vi "Begin.vi"(8 "error in (no error)":errorcluster, 10 "Settings":variant, 11 "Elevator Concrete in":refnum<class "Elevator Linear.lvclass">) -> (0 "error out":errorcluster, 3 "Elevator Concrete out":refnum<class "Elevator Linear.lvclass">)   [LabVIEW 2019, in "Elevator.lvlib" / "Elevator Linear.lvclass"]
doc: "This VI intializes the linear elevator."
uses:
  Elevator Linear.lvclass
  C:/Users/Public/Documents/2020InfinteRecharge/src robot/Classes/Elevator/Elevator.lvclass
  <vilib>/Rock Robotics/WPI/ThirdParty/Phoenix-LabVIEW/Motor Controller/Controls/CTRE_Phoenix_MotorControl_EnhancedMotorControllerConfigurables.ctl
  <vilib>/Rock Robotics/WPI/ThirdParty/Phoenix-LabVIEW/Motor Controller/Controls/CTRE_Phoenix_MotorControl_BaseConfigurables.ctl
  <vilib>/Rock Robotics/WPI/ThirdParty/Phoenix-LabVIEW/Motor Controller/Controls/CTRE_Phoenix_MotorControl_VelocityMeasurementPeriod.ctl
  <vilib>/Rock Robotics/WPI/ThirdParty/Phoenix-LabVIEW/Motor Controller/Controls/CTRE_Phoenix_MotorControl_SlotStructure.ctl
  <vilib>/Rock Robotics/WPI/ThirdParty/Phoenix-LabVIEW/Motor Controller/Controls/CTRE_Phoenix_MotorControl_FilterStruct.ctl
  <vilib>/Rock Robotics/WPI/ThirdParty/Phoenix-LabVIEW/Motor Controller/Controls/CTRE_Phoenix_MotorControl_RemoteSourceType.ctl
  <vilib>/Rock Robotics/WPI/ThirdParty/Phoenix-LabVIEW/Controls/CTRE_Phoenix_CustomParamConfiguration.ctl
  <vilib>/Rock Robotics/WPI/ThirdParty/Phoenix-LabVIEW/Motor Controller/Controls/CTRE_Phoenix_MotorControl_FeedbackDevice.ctl
  <vilib>/Rock Robotics/WPI/ThirdParty/Phoenix-LabVIEW/Motor Controller/Controls/CTRE_Phoenix_MotorControl_SensorTermFeedbackDevice_Enhanced.ctl
  <vilib>/Rock Robotics/WPI/ThirdParty/Phoenix-LabVIEW/Motor Controller/Controls/CTRE_Phoenix_MotorControl_LimitSwitchNormal.ctl
  <vilib>/Rock Robotics/WPI/ThirdParty/Phoenix-LabVIEW/Motor Controller/Controls/CTRE_Phoenix_MotorControl_LimitSwitchSource_Local.ctl
  Controls/Elevator Position.ctl
  Elevator Linear.lvclass/Elevator Linear.ctl
  Elevator.lvclass/Elevator.ctl
  Public Methods/Read Elevator Linear PID.vi
  Public Methods/Write Array.vi
  <vilib>/Rock Robotics/WPI/ThirdParty/Phoenix-LabVIEW/Motor Controller/Get/CTRE_Phoenix_MotorController_GetLimitSwitchStates.vi
  Elevator.lvclass
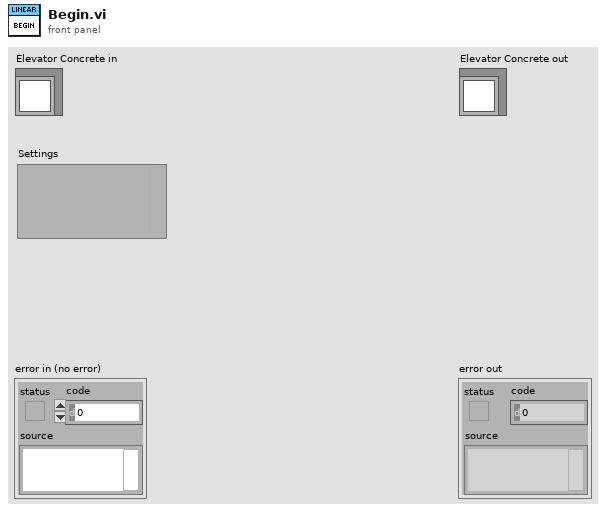
[diagram p1: front panel]
types:
  T1 = typedef "Elevator.lvlib/Elevator.lvclass/Elevator Position.ctl" = enum16{"CS, Cargo Ship Cargo", "C0, Cargo Ground", "C1, LV1 Cargo", "C2, LV2 Cargo", "C3, LV3 Cargo", "H0, LV1 Hatch", "H1, LV2 Hatch", "H2, LV3 Hatch"}
  T2 = enum16{"FollowerType_PercentOutput", "FollowerType_AuxOutput1"}
  T3 = typedef "CTRE_Phoenix_MotorControl_EnhancedMotorControllerConfigurables.ctl" = cluster{"Base Configurables":T4, "primaryPID":cluster{"selectedFeedbackCoefficient":dbl, "selectedFeedbackSensor":T10}, "auxiliaryPID":cluster{"selectedFeedbackCoefficient":dbl, "selectedFeedbackSensor":T10}, "sum0Term":T11, "sum1Term":T11, "diff0Term":T11, "diff1Term":T11, "forwardLimitSwitchNormal":T12, "reverseLimitSwitchNormal":T12, "forwardLimitSwitchDeviceID":i32, "reverseLimitSwitchDeviceID":i32, "forwardLimitSwitchSource":T13, "reverseLimitSwitchSource":T13, "peakCurrentLimit":i32, "peakCurrentDuration":i32, "continuousCurrentLimit":i32}
  T4 = typedef "CTRE_Phoenix_MotorControl_BaseConfigurables.ctl" = cluster{"openLoopRamp":dbl, "closedLoopRamp":dbl, "peakOutputForward":dbl, "peakOutputReverse":dbl, "nominalOutputForward":dbl, "nominalOutputReverse":dbl, "neutralDeadband":dbl, "voltageCompSaturation":dbl, "voltageMeasurementFilter":i32, "velocityMeasurementPeriod":T5, "velocityMeasurementWindow":i32, "forwardSoftLimitThreshold":i32, "reverseSoftLimitThreshold":i32, "forwardSoftLimitEnable":bool, "reverseSoftLimitEnable":bool, "slot0":T6, "slot1":T6, "slot2":T6, "slot3":T6, "auxPIDPolarity":bool, "remoteFilter0":T7, "remoteFilter1":T7, "motionCruiseVelocity":i32, "motionAcceleration":i32, "motionProfileTrajectoryPeriod":i32, "feedbackNotContinuous":bool, "remoteSensorClosedLoopDisableNeutralOnLOS":bool, "clearPositionOnLimitF":bool, "clearPositionOnLimitR":bool, "clearPositionOnQuadIdx":bool, "limitSwitchDisableNeutralOnLOS":bool, "softLimitDisableNeutralOnLOS":bool, "pulseWidthPeriod_EdgesPerRot":i32, "pulseWidthPeriod_FilterWindowSz":i32, "customParam":T9, "trajectoryInterpolationEnable":bool}
  T5 = typedef "CTRE_Phoenix_MotorControl_VelocityMeasurementPeriod.ctl" = u16
  T6 = typedef "CTRE_Phoenix_MotorControl_SlotStructure.ctl" = cluster{"P":dbl, "I":dbl, "D":dbl, "F":dbl, "integralZone":dbl, "allowableClosedLoopError":i32, "maxIntegralAccumulator":dbl, "closedLoopPeakOutput":dbl, "closedLoopPeriod":i32}
  T7 = typedef "CTRE_Phoenix_MotorControl_FilterStruct.ctl" = cluster{"remoteSensorDeviceID":u8, "remoteSensorSource":T8}
  T8 = typedef "CTRE_Phoenix_MotorControl_RemoteSourceType.ctl" = enum16{"Off", "Talon SRX Selected Sensor", "Pigeon IMU Yaw", "Pigeon IMU Pitch", "Pigeon IMU Roll", "CANifier Quadrature", "CANifier PWM Input 0", "CANifier PWM Input 1", "CANifier PWM Input 2", "CANifier PWM Input 3", "Gadgeteer Pigeon Yaw", "Gadgeteer Pigeon Pitch", "Gadgeteer Pigeon Roll", "CANCoder"}
  T9 = typedef "CTRE_Phoenix_CustomParamConfiguration.ctl" = cluster{"customParam0":i32, "customParam1":i32}
  T10 = typedef "CTRE_Phoenix_MotorControl_FeedbackDevice.ctl" = i8
  T11 = typedef "CTRE_Phoenix_MotorControl_SensorTermFeedbackDevice_Enhanced.ctl" = i8
  T12 = typedef "CTRE_Phoenix_MotorControl_LimitSwitchNormal.ctl" = enum16{"Normally Open", "Normally Closed", "Disabled"}
  T13 = typedef "CTRE_Phoenix_MotorControl_LimitSwitchSource_Local.ctl" = enum16{"Feedback Connector", "Remote Talon SRX", "Remote CANifier", "Deactivated"}
  T14 = typedef "Elevator.lvlib/Elevator.lvclass/Elevator Constants.ctl" = cluster{"Arm Motion Magic Max Velocity":u32, "Arm Motion Magic Max Acceleration":u32, "Wrist Motion Magic Max Velocity":u32, "Wrist Motion Magic Max Acceleration":u32, "Elevator Linear Motion Magic Max Velocity":u32, "Elevator Linear Motion Magic Max Acceleration":u32, "Arm Gear Ratio":dbl, "Wrist Gear Ratio":dbl, "Elevator Linear Gear Ratio":dbl, "Arm Encoder ABS Value":i32, "Wrist Encoder ABS Value":i32}
  T15 = typedef "Elevator.lvlib/Elevator.lvclass/Elevator IDs.ctl" = cluster{"Wrist":u8, "Left Master":u8, "Left Slave":u8, "Right Master":u8, "Right Slave":u8, "Vacumm Pump 1":u8, "Vacumm Pump 2":u8, "Elevator Linear Master":u8, "Elevator Linear Slave":u8}
  T16 = typedef "WPI_MotorControlDeviceRef.ctl" = cluster{"DeviceStatus":errorcluster, "Type":T17, "PWM":cluster{"PWM Channel":T18, "DeadBand":T19}, "CAN":cluster{"Device Number":u8, "SetOutput VI Ref":variant, "GetOutput VI Ref":variant, "Enable VI Ref":variant, "Disable VI Ref":variant, "Data":variant}, "Invert":bool, "DIO PWM":cluster{"PWM \"Enable\" Channel":T18, "DIOChannel":T20, "PWM Rate":dbl}}
  T17 = typedef "WPI_MotorControlType.ctl" = enum16{"PWM", "CAN", "DIO PWM"}
  T18 = typedef "FPGA_DIOPWMChannel.ctl" = enum8{"PWM 0", "PWM 1", "PWM 2", "PWM 3", "PWM 4", "PWM 5", "PWM 6", "PWM 7", "PWM 8", "PWM 9", "PWM MXP 0", "PWM MXP 1", "PWM MXP 2", "PWM MXP 3", "PWM MXP 4", "PWM MXP 5", "PWM MXP 6", "PWM MXP 7", "PWM MXP 8", "PWM MXP 9", "Invalid"}
  T19 = typedef "WPI_PWMDeadband.ctl" = cluster{"Name":string, "maxPositivePwm":i32, "minPositivePwm":i32, "centerPwm":i32, "maxNegativePwm":i32, "minNegativePwm":i32, "angularRange":u16}
  T20 = typedef "FPGA_DIOChannel.ctl" = enum8{"DIO 0", "DIO 1", "DIO 2", "DIO 3", "DIO 4", "DIO 5", "DIO 6", "DIO 7", "DIO 8", "DIO 9", "DIO MXP 0", "DIO MXP 1", "DIO MXP 2", "DIO MXP 3", "DIO MXP 4", "DIO MXP 5", "DIO MXP 6", "DIO MXP 7", "DIO MXP 8", "DIO MXP 9", "DIO MXP 10", "DIO MXP 11", "DIO MXP 12", "DIO MXP 13", "DIO MXP 14", "DIO MXP 15", "SPI Port CS1", "SPI Port CS2", "SPI Port CS3", "SPI Port MISO", "SPI Port MOSI", "Invalid"}
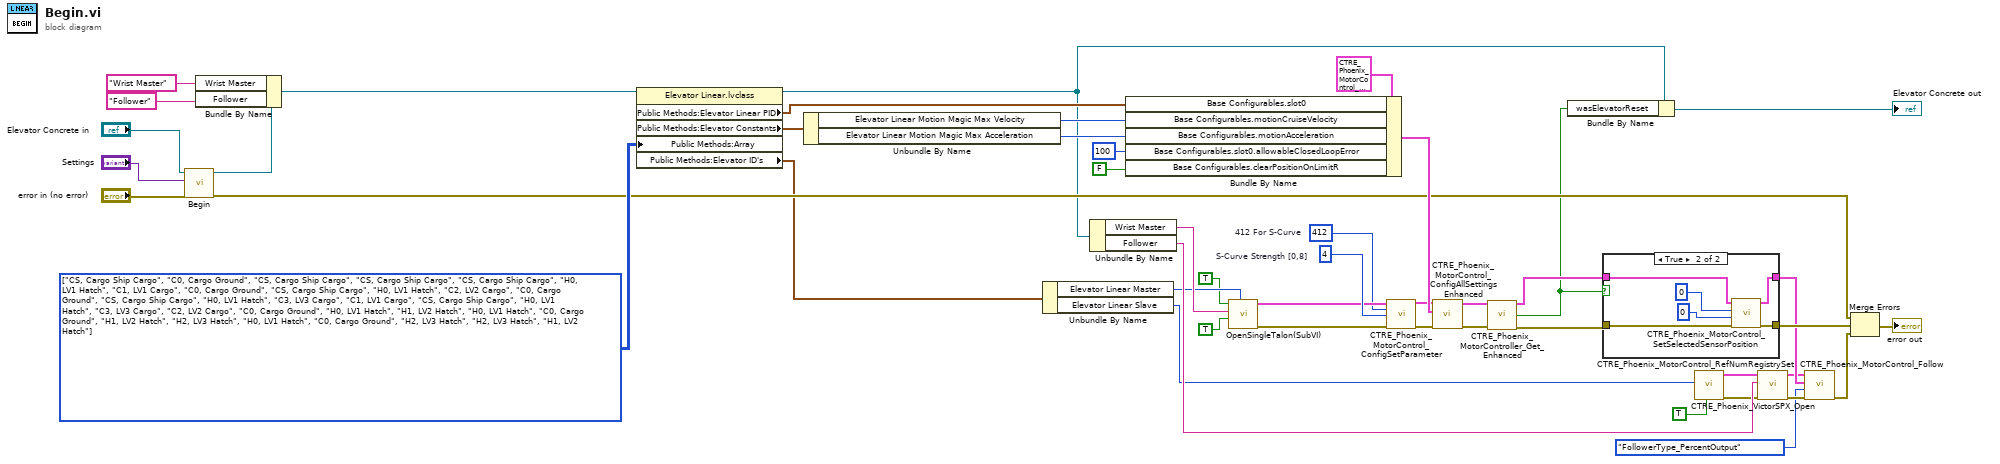
[diagram p0: block diagram]
diagram:
  w17 = T1[][] [[enum."CS, Cargo Ship Cargo", enum."C0, Cargo Ground", enum."CS, Cargo Ship Cargo", enum."CS, Cargo Ship Cargo"], [enum."CS, Cargo Ship Cargo", enum."H0, LV1 Hatch", enum."C1, LV1 Cargo", enum."C0, Cargo Ground"], [enum."CS, Cargo Ship Cargo", enum."H0, LV1 Hatch", enum."C2, LV2 Cargo", enum."C0, Cargo Ground"], [enum."CS, Cargo Ship Cargo", enum."H0, LV1 Hatch", enum."C3, LV3 Cargo", enum."C1, LV1 Cargo"], [enum."CS, Cargo Ship Cargo", enum."H0, LV1 Hatch", enum."C3, LV3 Cargo", enum."C2, LV2 Cargo"], [enum."C0, Cargo Ground", enum."H0, LV1 Hatch", enum."H1, LV2 Hatch", enum."H0, LV1 Hatch"], [enum."C0, Cargo Ground", enum."H1, LV2 Hatch", enum."H2, LV3 Hatch", enum."H0, LV1 Hatch"], [enum."C0, Cargo Ground", enum."H2, LV3 Hatch", enum."H2, LV3 Hatch", enum."H1, LV2 Hatch"]] items=["CS, Cargo Ship Cargo", "C0, Cargo Ground", "C1, LV1 Cargo", "C2, LV2 Cargo", "C3, LV3 Cargo", "H0, LV1 Hatch", "H1, LV2 Hatch", "H2, LV3 Hatch"] ("Array")
  w32 = u32 412  # 412 For S-Curve
  w37 = 4  # S-Curve Strength [0,8]
  n1 = call-parent "Begin.vi"("error in (no error)"="error in (no error)", "Settings"="Settings", "Elevator in"="Elevator Concrete in") -> ("error out"=w12:errorcluster, "Elevator out"=w14:refnum<class "Elevator Linear.lvclass">)  [unwired: 7 in]
  n2 = Bundle By Name(cluster=w14, "Wrist Master"="Wrist Master", "Follower"="Follower") -> (w28:refnum<class "Elevator Linear.lvclass">)
  n3 = property class="Elevator Linear.lvclass"(reference=w28, "Public Methods:Array"=w17) -> (reference out=w4:refnum<class "Elevator Linear.lvclass">, "Public Methods:Elevator Linear PID"=w11:T6, "Public Methods:Elevator Constants"=w18:T14, "Public Methods:Elevator ID's"=w5:T15)  [unwired: 1 in, 1 out]
  n4 = Unbundle By Name(w18) -> ("Elevator Linear Motion Magic Max Velocity"=w41:u32, "Elevator Linear Motion Magic Max Acceleration"=w40:u32)
  n5 = Unbundle By Name(w5) -> ("Elevator Linear Master"=w38:u8, "Elevator Linear Slave"=w39:u8)
  n6 = Unbundle By Name(w4) -> ("Wrist Master"=w46:string, "Follower"=w45:string)
  n7 = Bundle By Name(cluster=T3 {"Base Configurables"={"openLoopRamp"=0.0, "closedLoopRamp"=0.0, "peakOutputForward"=1.0, "peakOutputReverse"=-1.0, "nominalOutputForward"=0.0, "nominalOutputReverse"=0.0, "neutralDeadband"=0.04, "voltageCompSaturation"=0.0, "voltageMeasurementFilter"=32, "velocityMeasurementPeriod"=100, "velocityMeasurementWindow"=64, "forwardSoftLimitThreshold"=0, "reverseSoftLimitThreshold"=0, "forwardSoftLimitEnable"=FALSE, "reverseSoftLimitEnable"=FALSE, "slot0"={"P"=0.0, "I"=0.0, "D"=0.0, "F"=0.0, "integralZone"=0.0, "allowableClosedLoopError"=0, "maxIntegralAccumulator"=0.0, "closedLoopPeakOutput"=1.0, "closedLoopPeriod"=1}, "slot1"={"P"=0.0, "I"=0.0, "D"=0.0, "F"=0.0, "integralZone"=0.0, "allowableClosedLoopError"=0, "maxIntegralAccumulator"=0.0, "closedLoopPeakOutput"=1.0, "closedLoopPeriod"=1}, "slot2"={"P"=0.0, "I"=0.0, "D"=0.0, "F"=0.0, "integralZone"=0.0, "allowableClosedLoopError"=0, "maxIntegralAccumulator"=0.0, "closedLoopPeakOutput"=1.0, "closedLoopPeriod"=1}, "slot3"={"P"=0.0, "I"=0.0, "D"=0.0, "F"=0.0, "integralZone"=0.0, "allowableClosedLoopError"=0, "maxIntegralAccumulator"=0.0, "closedLoopPeakOutput"=1.0, "closedLoopPeriod"=1}, "auxPIDPolarity"=FALSE, "remoteFilter0"={"remoteSensorDeviceID"=0, "remoteSensorSource"=enum."Off"}, "remoteFilter1"={"remoteSensorDeviceID"=0, "remoteSensorSource"=enum."Off"}, "motionCruiseVelocity"=0, "motionAcceleration"=0, "motionProfileTrajectoryPeriod"=0, "feedbackNotContinuous"=FALSE, "remoteSensorClosedLoopDisableNeutralOnLOS"=FALSE, "clearPositionOnLimitF"=FALSE, "clearPositionOnLimitR"=FALSE, "clearPositionOnQuadIdx"=FALSE, "limitSwitchDisableNeutralOnLOS"=FALSE, "softLimitDisableNeutralOnLOS"=FALSE, "pulseWidthPeriod_EdgesPerRot"=1, "pulseWidthPeriod_FilterWindowSz"=1, "customParam"={"customParam0"=0, "customParam1"=0}, "trajectoryInterpolationEnable"=TRUE}, "primaryPID"={"selectedFeedbackCoefficient"=1.0, "selectedFeedbackSensor"=0}, "auxiliaryPID"={"selectedFeedbackCoefficient"=1.0, "selectedFeedbackSensor"=0}, "sum0Term"=0, "sum1Term"=0, "diff0Term"=0, "diff1Term"=0, "forwardLimitSwitchNormal"=enum."Normally Open", "reverseLimitSwitchNormal"=enum."Normally Open", "forwardLimitSwitchDeviceID"=0, "reverseLimitSwitchDeviceID"=0, "forwardLimitSwitchSource"=enum."Feedback Connector", "reverseLimitSwitchSource"=enum."Feedback Connector", "peakCurrentLimit"=1, "peakCurrentDuration"=1, "continuousCurrentLimit"=1} ("Enhanced Motor Controller Configurables"), "Base Configurables.slot0"=w11, "Base Configurables.motionCruiseVelocity"=w41, "Base Configurables.motionAcceleration"=w40, "Base Configurables.slot0.allowableClosedLoopError"=100, "Base Configurables.clearPositionOnLimitR"=FALSE) -> (w43:T3)
  n8 = call "OpenSingleTalon(SubVI).vi"("can_id"=w38, "sensor_phase"=TRUE, "refnum name"=w46, "invert"=TRUE) -> ("error out"=w34:errorcluster, "PhoenixMotorControlDevRef"=w36:T16)  [unwired: 6 in]
  n9 = call <vilib>:"CTRE_Phoenix_MotorControl_ConfigSetParameter.vi"("PhoenixMotorControlDevRef"=w36, "Parameter"=w32, "value"=w37, "error in (no error)"=w34) -> ("PhoenixMotorControlDevRef"=w35:T16, "error out"=w33:errorcluster)  [unwired: 10 in]
  n10 = call <vilib>:"CTRE_Phoenix_MotorControl_ConfigAllSettingsEnhanced.vi"("error in (no error)"=w33, "Enhanced Motor Controller Configurables"=w43, "PhoenixMotorControlDevRef"=w35) -> ("error out"=w2:errorcluster, "PhoenixMotorControlDevRef"=w10:T16)  [unwired: 7 in]
  n11 = call-poly <vilib>:"CTRE_Phoenix_MotorController_Get_Enhanced.vi"("PhoenixMotorControlDevRef"=w10, "error in"=w2) -> ("PhoenixMotorControlDevRef"=w9:T16, "Reverse Limit Closed?"=w7:bool, "error out"=w1:errorcluster)  [unwired: 10 in, 1 out]
  n12 = Bundle By Name(cluster=w4, "wasElevatorReset"=w7) -> (→"Elevator Concrete out":refnum<class "Elevator Linear.lvclass">)
  n13 = case shown="True" w7 {
    tunnel: w1 -> [w48 w55]
    tunnel: [w48 w52] -> w30
    tunnel: [w49 w51] -> w29
    tunnel: w9 -> [w49 w50]
    frame False {
    }
    frame True {
      n14 = call <vilib>:"CTRE_Phoenix_MotorControl_SetSelectedSensorPosition.vi"("error in (no error)"=w55, "pidLoopIdx"=0 ("New Sensor Position"), "New Sensor Position"=0, "PhoenixMotorControlDevRef"=w50) -> ("error out"=w52:errorcluster, "PhoenixMotorControlDevRef"=w51:T16)  [unwired: 6 in]
    }
  }
  n15 = call <vilib>:"CTRE_Phoenix_VictorSPX_Open.vi"("Invert"=TRUE, "Device Number"=w39) -> ("error out"=w25:errorcluster, "CAN Talon SRX Ref"=w24:T16)  [unwired: 8 in]
  n16 = call <vilib>:"CTRE_Phoenix_MotorControl_RefNumRegistrySet.vi"("error in (no error)"=w25, "refnum name"=w45, "PhoenixMotorControlDevRef"=w24) -> ("error out"=w22:errorcluster, "PhoenixMotorControlDevRef"=w23:T16)  [unwired: 7 in]
  n17 = call <vilib>:"CTRE_Phoenix_MotorControl_Follow.vi"("error in (no error)"=w22, "FollowerType"=T2."FollowerType_PercentOutput", "Master Controller to Follow"=w29, "PhoenixMotorControlDevRef"=w23) -> ("error out"=w31:errorcluster)  [unwired: 6 in, 1 out]
  n18 = Merge Errors(w12, w30, w31) -> (→"error out":errorcluster)
